vi "Get Image Data.vi"(11 "Animation":enum16{"Green Bars"}(ring)) -> (3 "Frame Data":T1[](array[typedef]))   [LabVIEW 2011, in "LVH-Toolbox.lvlib" / "LVH-SystemTools.lvlib"]
uses:
  LVH-SystemTools.lvlib
  <vilib>/picture/picture.llb/imagedata.ctl
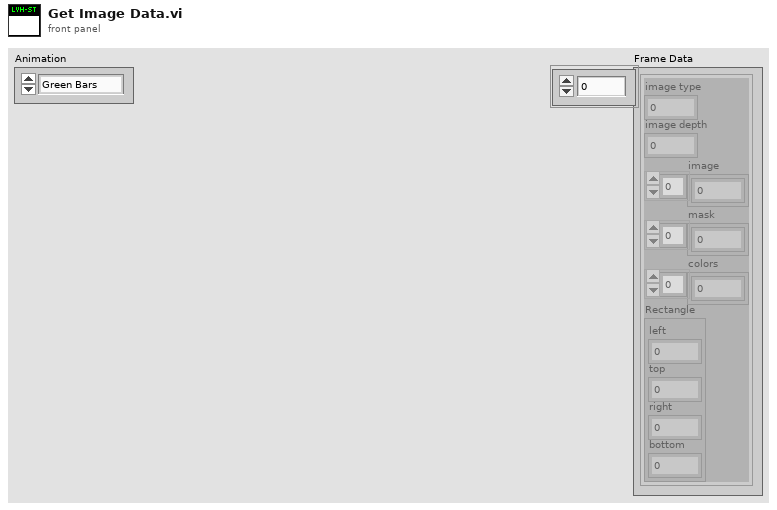
[diagram p1: front panel]
types:
  T1 = typedef "imagedata.ctl" = cluster{"image type":i32, "image depth":i32, "image":u8[], "mask":u8[], "colors":u32[], "Rectangle":cluster{"left":i16, "top":i16, "right":i16, "bottom":i16}}
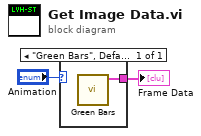
[diagram p0: block diagram]
diagram:
  n1 = case shown="\"Green Bars\", Default" "Animation" {
    tunnel: [w3] -> w1
    frame "Green Bars", Default {
      n2 = call "Green Bars.vi"() -> ("Green Bars"=w3:T1[])  [unwired: 11 in]
    }
  }
  "Frame Data" <- w1
